vi "UDP Data Link - RTMs - Export to XML.vi"(8 "error in (no error)":errorcluster, 11 "Node Ptr":u64 format="%.0x") -> (0 "error out":errorcluster)   [LabVIEW 2015, in "UDP Data Link System Explorer.lvlib"]
uses:
  UDP Data Link System Explorer.lvlib
  <vilib>/NI Veristand/Custom Device Tools/Custom Device Utility Library/Custom Device Utility Library.lvlib
panel:
  in  "Tag":string
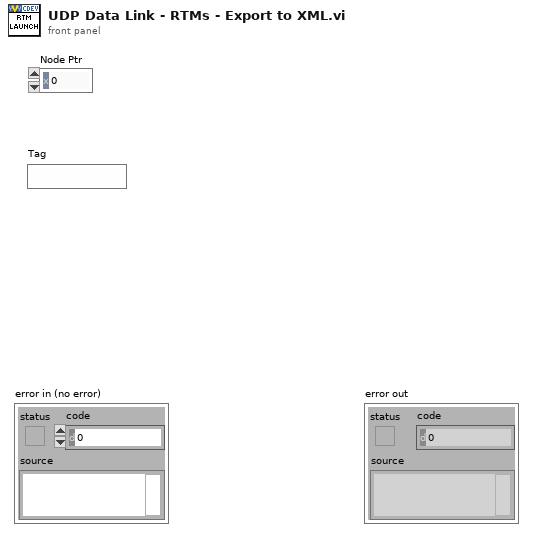
[diagram p1: front panel]
types:
  T1 = typedef "Custom Device API.lvlib/Custom Device Item Ref.ctl" = u64
  T2 = typedef "UDP Data Link System Explorer.lvlib/UDP Data Link - TypeDefs - XML Header Data.ctl" = cluster{"Revision (\"Major.Minor.Fix.Build\")":string, "Creation Date (\"yyyy-mm-dd\")":string, "Controller Name":string}
  T3 = typedef "UDP Data Link System Explorer.lvlib/UDP Data Link - TypeDefs - XML Group.ctl" = cluster{"Freq":i32, "Tx Channels":T4[], "Rx Channels":T4[]}
  T4 = typedef "UDP Data Link System Explorer.lvlib/UDP Data Link - TypeDefs - XML Channel.ctl" = cluster{"Channel Name":string, "Data Type":u16, "Description":string, "Unit":string}
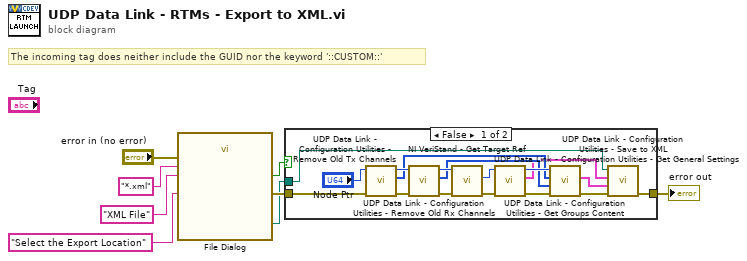
[diagram p0: block diagram]
diagram:
  # "The incoming tag does neither include the GUID nor the keyword '::CUSTOM::'"
  n1 = call "File Dialog"("prompt"="Select the Export Location", "error in"="error in (no error)", "pattern (all files)"="*.xml", "pattern label"="XML File") -> ("selected path"=w2:path, "cancelled"=w4:bool, "error out"=w3:errorcluster)  [unwired: 8 in, 1 out]
  n2 = case shown="False" w4 {
    tunnel: w3 -> [w19 w26]
    tunnel: w2 -> [w16 _]
    tunnel: [w9 w26] -> w1
    frame False {
      n3 = call "UDP Data Link - Configuration Utilities - Remove Old Tx Channels.vi"("error in (no error)"=w19, "Device Item Ref in"="Node Ptr") -> ("error out"=w21:errorcluster, "Tx Dependent Refs"=w15:T1[], "Device Item Ref out"=w18:T1)  [unwired: 7 in]
      n4 = call "UDP Data Link - Configuration Utilities - Remove Old Rx Channels.vi"("error in (no error)"=w21, "Device Item Ref in"=w18) -> ("error out"=w13:errorcluster, "Rx Dependent Refs"=w14:T1[], "Device Item Ref out"=w17:T1)  [unwired: 7 in]
      n5 = call <vilib>:"NI VeriStand - Get Target Ref.vi"("error in"=w13, "Item Ref in"=w17) -> ("error out"=w24:errorcluster, "Target Ref"=w23:T1)  [unwired: 6 in, 2 out]
      n6 = call "UDP Data Link - Configuration Utilities - Get General Settings.vi"("error in (no error)"=w24, "Target Ref in"=w23) -> ("error out"=w25:errorcluster, "XML Header Data"=w12:T2, "Target Ref out"=w22:T1)  [unwired: 7 in]
      n7 = call "UDP Data Link - Configuration Utilities - Get Groups Content.vi"("error in (no error)"=w25, "Rx"=w14, "Tx"=w15, "Target Ref In"=w22) -> ("error IO"=w10:errorcluster, "Groups"=w11:T3[])  [unwired: 5 in, 1 out]
      n8 = call "UDP Data Link - Configuration Utilities - Save to XML.vi"("error in"=w10, "Channel Groups"=w11, "XML Header Data"=w12, "XML File Path"=w16) -> ("error out"=w9:errorcluster)  [unwired: 7 in]
    }
    frame True {
    }
  }
  "error out" <- w1
